vi "Access2DArray.vi"(4 "Sequence Context":refnum<k7>) -> (0 "error out":errorcluster)   [LabVIEW 2011]
doc: "Reads the two dimensional array data from the local variable using the TestStand API and displays it in a graph."
panel:
  in  "OK":bool
  out "Array of Data":dbl[][](graph)
  # "Array Data"
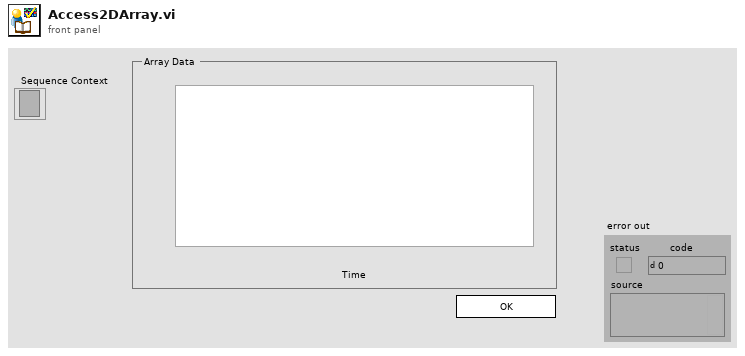
[diagram p1: front panel]
types:
  T1 = typedef "TestStand - Status Monitor.ctl" = cluster{"Sequence Context":refnum<k7>, "Execution":refnum<k7>, "Termination Monitor":refnum<k7>}
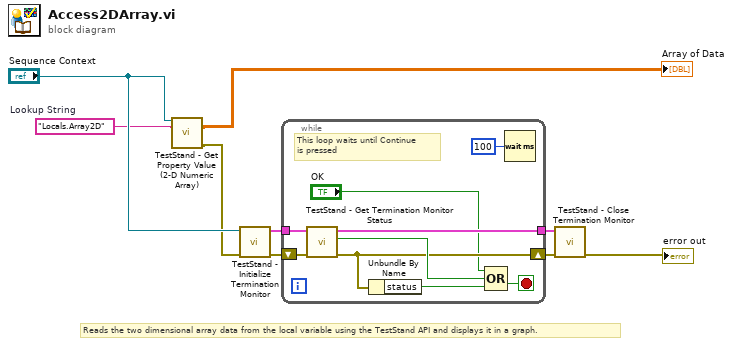
[diagram p0: block diagram]
diagram:
  w2 = "Locals.Array2D"  # Lookup String
  # "Reads the two dimensional array data from the local variable using the TestStand API and displays it in a graph."
  n1 = call "TestStand - Get Property Value (2-D Numeric Array).vi"("Sequence Context In"="Sequence Context", "Lookup String"=w2) -> ("Value"=→"Array of Data":dbl[][], "error out"=w1:errorcluster)  [unwired: 2 in, 10 out]
  n2 = call <vilib>:"TestStand - Initialize Termination Monitor.vi"("error in (no error)"=w1, "Sequence Context In"="Sequence Context") -> ("error out"=w7:errorcluster, "Status Monitor Out"=w9:T1)  [unwired: 8 out]
  n3 = while {
    shift-left: w7 -> [w16]
    shift-right: [w13] -> w6
    tunnel: [w17] -> w8
    tunnel: w9 -> [w18]
    stop <- w15 stop-if-true
    # "This loop waits until Continue \nis pressed"
    n4 = call <vilib>:"TestStand - Get Termination Monitor Status.vi"("error in (no error)"=w16, "Status Monitor In"=w18) -> ("error out"=w13:errorcluster, "Terminating or Aborting"=w14:bool, "Status Monitor Out"=w17:T1)  [unwired: 7 out]
    n5 = Unbundle By Name(w13) -> ("status"=w12:bool)
    n6 = Compound Arithmetic op=OR("OK", w14, w12) -> (w15:bool)
    n7 = Wait (ms)(milliseconds to wait=u32 100) -> ()  [unwired: 1 out]
  }
  n8 = call <vilib>:"TestStand - Close Termination Monitor.vi"("error in (no error)"=w6, "Status Monitor In"=w8) -> ("error out"=→"error out":errorcluster)  [unwired: 9 out]
